vi "Normalize by DPI.vi"(8 "error in (no error)":errorcluster, 10 "window rect":T1, 11 "window refnum (NaWR)":T2) -> (0 "error out":errorcluster, 2 "normalized window rect":T1, 3 "window refnum out":T2)   [LabVIEW 2020, in "MacroAssert.lvlib" / "Win Util.lvlib"]
uses:
  Win Util.lvlib
  System.Windows.Forms
  System.Drawing
  Window Refnum.ctl
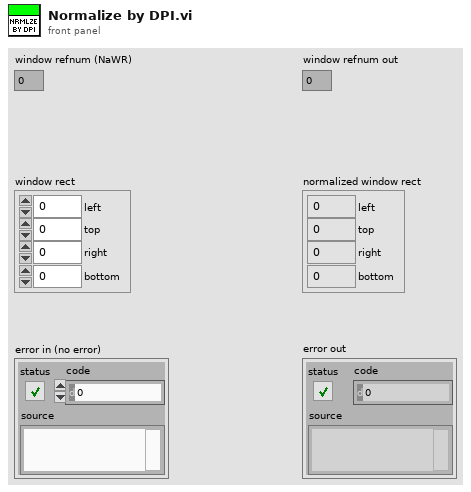
[diagram p1: front panel]
types:
  T1 = cluster{"left":i16, "top":i16, "right":i16, "bottom":i16}
  T2 = typedef "MacroAssert.lvlib/Win Util.lvlib/Window Refnum.ctl" = u64
  T3 = cluster{"Left":i32, "Top":i32, "Left":i32, "Top":i32}
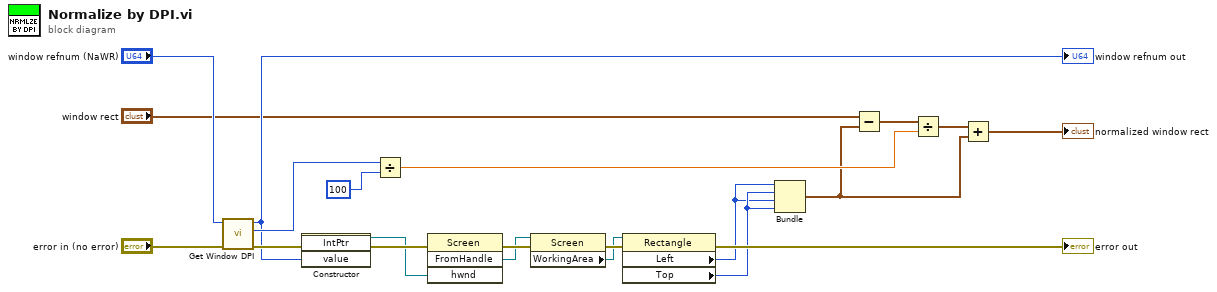
[diagram p0: block diagram]
diagram:
  n1 = call "Get Window DPI.vi"("error in"="error in (no error)", "window refnum in"="window refnum (NaWR)") -> ("error out"=w17:errorcluster, "DPI"=w9:i32, "window refnum out"=w7:T2)  [unwired: 7 in]
  "window refnum out" <- w7
  n2 = constructor class="IntPtr"(error in=w17, "value"=w7) -> (reference out=w13:refnum<k24>, error out=w21:errorcluster)  [unwired: 2 in, 2 out]
  n3 = Divide(x=w9, y=100) -> (x/y=w5:dbl)
  n4 = invoke class="Screen" method="FromHandle"(error in=w21, "hwnd"=w13) -> (error out=w20:errorcluster, "FromHandle"=w15:refnum<k24>)  [unwired: 2 in, 2 out]
  n5 = property class="Screen"(reference=w15, error in=w20) -> (error out=w19:errorcluster, "WorkingArea"=w14:refnum<k24>)  [unwired: 1 out]
  n6 = property class="Rectangle"(reference=w14, error in=w19) -> (error out=→"error out":errorcluster, "Left"=w11:i32, "Top"=w12:i32)  [unwired: 1 out]
  n7 = Bundle("Left"=w11, "Top"=w12, "Left"=w11, "Top"=w12) -> (w1:T3)  [unwired: 1 in]
  n8 = Subtract(x="window rect", y=w1) -> (x-y=w6:cluster{i32, i32, i32, i32})
  n9 = Divide(x=w6, y=w5) -> (x/y=w4:cluster{dbl, dbl, dbl, dbl})
  n10 = Add(x=w4, y=w1) -> (x+y=→"normalized window rect":cluster{dbl, dbl, dbl, dbl})
